vi "mobileyepaser.vi"() -> (2 "headway time":dbl)   [LabVIEW 2015]
uses:
  G_LCM.vi
  G_SEN.vi
panel:
  out "Array":dbl[][](array[numeric])
  out "vel":dbl
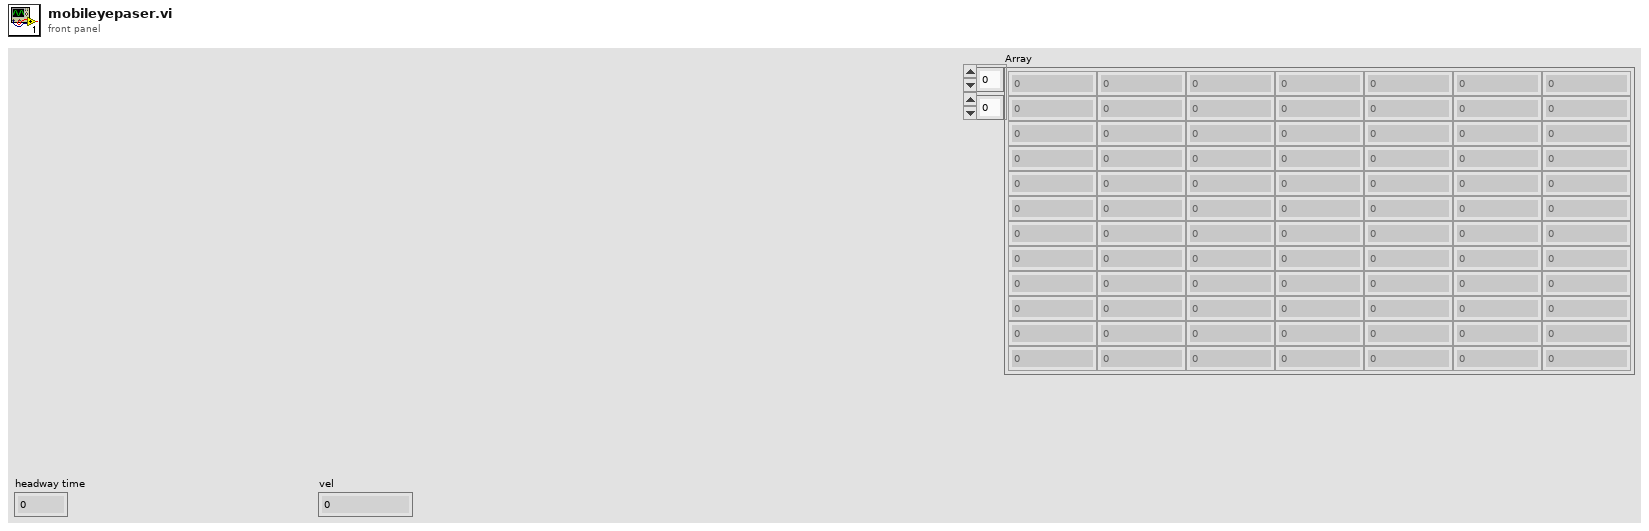
[diagram p1: front panel]
types:
  T1 = cluster{"hash":i64, "sys time":i64, "mobileye":u8[]}
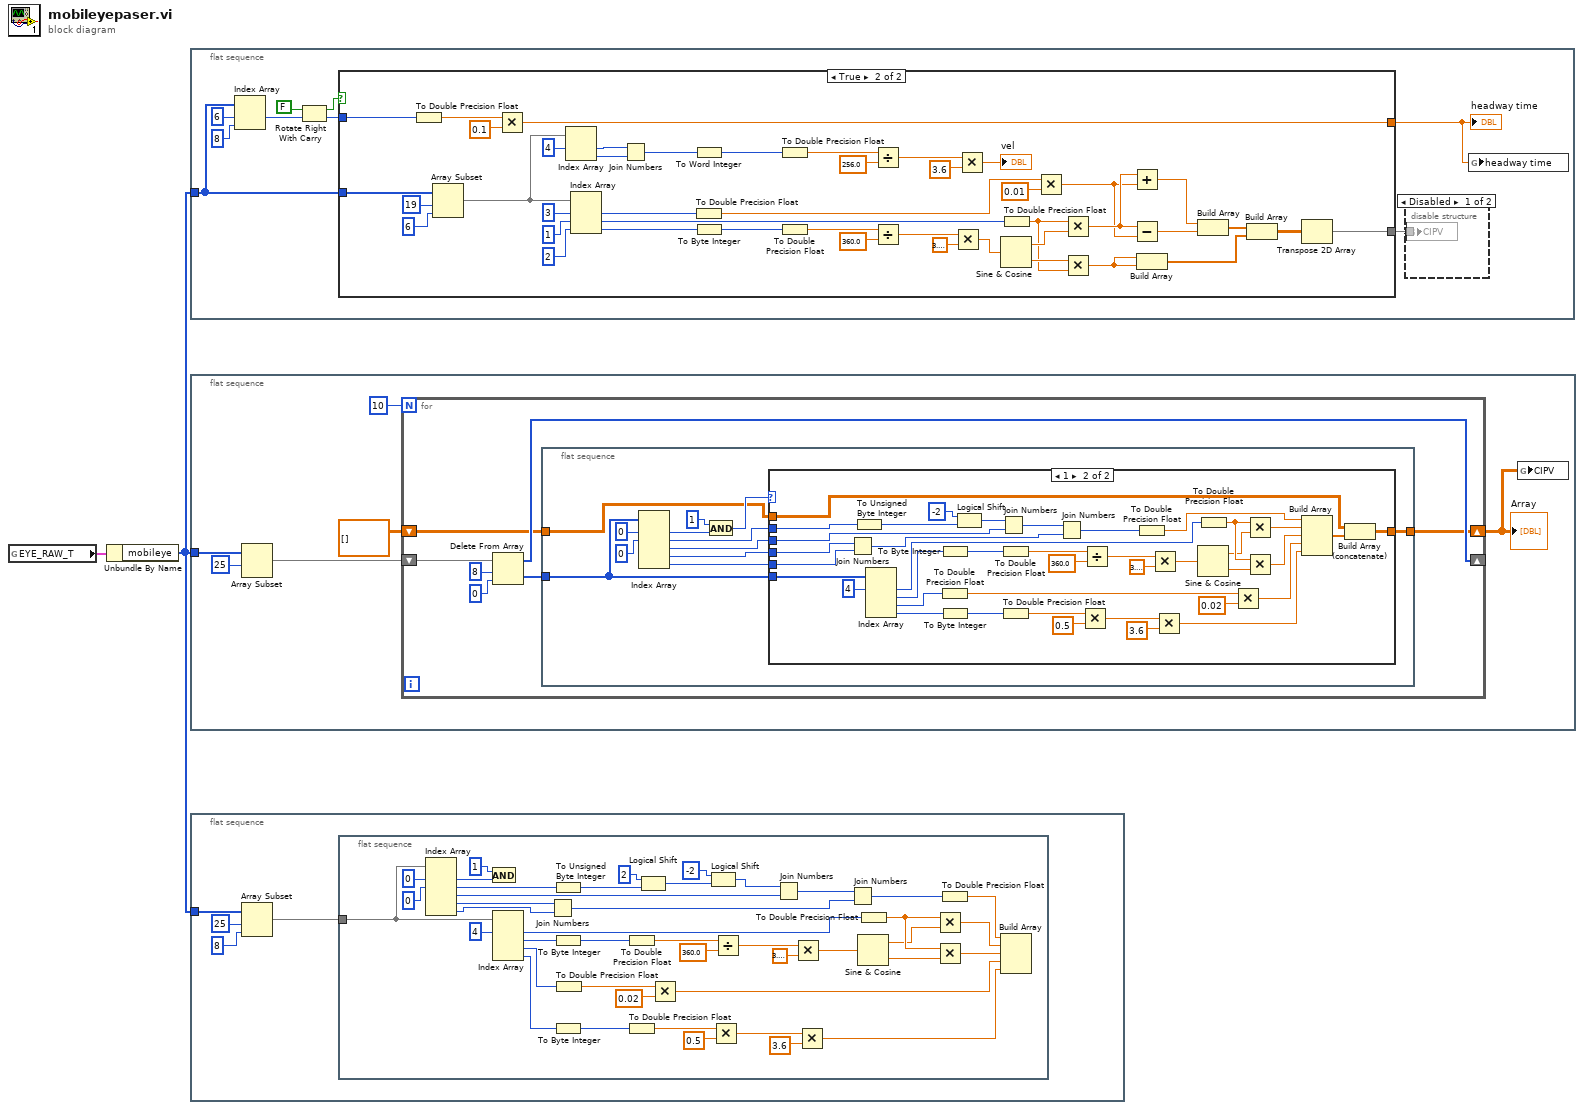
[diagram p0: block diagram]
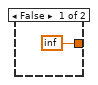
[diagram p4: hidden frame]
diagram:
  n1 = global read "G_LCM.vi" "EYE_RAW_T"() -> (w2:T1)
  n2 = Unbundle By Name(w2) -> ("mobileye"=w1:u8[])
  n3 = flat-sequence {
    tunnel: w1 -> [w5]
    frame #0 {
      n4 = Index Array(array=w5, index #1=6 ("index"), index #2=8 ("index")) -> (element #1=w9:u8)  [unwired: 1 out]
      n5 = Rotate Right With Carry(2:w9, 3:FALSE ("carry")) -> (0:w7:u8, 1:w6:bool)
      n6 = case shown="True" w6 {
        tunnel: w7 -> [_ w28]
        tunnel: [inf w27] -> w3
        tunnel: w5 -> [_ w57]
        tunnel: [_ w31] -> w4
        frame False {
        }
        frame True {
          n7 = To Double Precision Float(number=w28) -> (double precision float=w30:dbl)
          n8 = Array Subset(array=w57, index=19, length=6) -> (w26:u8[])
          n9 = Multiply(x=w30, y=0.1) -> (x*y=w27:dbl)
          n10 = Index Array(array=w26, index #1=4 ("index")) -> (element #1=w48:u8, element #2=w47:u8)  [unwired: 1 in]
          n11 = Index Array(array=w26, index #1=3 ("index"), index #2=1 ("index"), index #3=2 ("index")) -> (element #1=w24:u8, element #2=w18:u8, element #3=w22:u8)
          n12 = Join Numbers(hi=w48, lo=w47) -> ((hi.lo)=w16:u16)
          n13 = To Word Integer(number=w16) -> (16bit integer=w15:i16)
          n14 = To Double Precision Float(number=w24) -> (double precision float=w23:dbl)
          n15 = To Byte Integer(number=w22) -> (8bit integer=w21:i8)
          n16 = To Double Precision Float(number=w15) -> (double precision float=w46:dbl)
          n17 = To Double Precision Float(number=w21) -> (double precision float=w20:dbl)
          n18 = Divide(x=w46, y=256.0) -> (x/y=w44:dbl)
          n19 = Divide(x=w20, y=360.0) -> (x/y=w52:dbl)
          n20 = Multiply(x=w52, y=3.141592653589793) -> (x*y=w42:dbl)
          n21 = Multiply(x=w44, y=3.6) -> (x*y=→"vel":dbl)
          n22 = Sine & Cosine(0:w42) -> (1:w41:dbl, 2:w40:dbl)
          n23 = To Double Precision Float(number=w18) -> (double precision float=w17:dbl)
          n24 = Multiply(x=w23, y=0.01) -> (x*y=w38:dbl)
          n25 = Multiply(x=w17, y=w41) -> (x*y=w39:dbl)
          n26 = Multiply(x=w40, y=w17) -> (x*y=w35:dbl)
          n27 = Add(x=w39, y=w38) -> (x+y=w37:dbl)
          n28 = Subtract(x=w39, y=w38) -> (x-y=w36:dbl)
          n29 = Build Array(w35, w35) -> (w33:dbl[])
          n30 = Build Array(w37, w36) -> (w34:dbl[])
          n31 = Build Array(w34, w33) -> (w32:dbl[][])
          n32 = Transpose 2D Array(2D array=w32) -> (transposed array=w31:dbl[][])
        }
      }
      "headway time" <- w3
      n33 = disable-structure shown="Disabled" {
        disable-tunnel: w4 -> [w12 _]
        frame Disabled {
          n34 = global write "G_SEN.vi" "CIPV"(w12) -> ()
        }
        frame Enabled {
        }
      }
      n35 = global write "G_SEN.vi" "headway time"(w3) -> ()
    }
  }
  n36 = flat-sequence {
    tunnel: w1 -> [w63]
    frame #0 {
      n37 = Array Subset(array=w63, index=25) -> (w61:u8[])  [unwired: 1 in]
      n38 = for {
        N: 10 -> [_]
        shift-right: [w69] -> _
        shift-left: w61 -> [w70]
        shift-right: [w65] -> w58
        shift-left: dbl[][] [] -> [w64]
        n39 = Delete From Array(array=w70, length=8, index=0) -> (deleted portion=w66:u8[], array with subset deleted=w69:u8[])
        n40 = flat-sequence {
          tunnel: w66 -> [w82]
          tunnel: [w72] -> w65
          tunnel: w64 -> [w71]
          frame #0 {
            n41 = Index Array(array=w82, index #1=0 ("index"), index #2=0 ("index")) -> (element #1=w74:u8, element #2=w80:u8, element #3=w79:u8, element #4=w78:u8, element #5=w77:u8)  [unwired: 3 in]
            n42 = And(x=u8 1 ("y"), y=w74) -> (x .and. y?=w73:u8)
            n43 = case shown="1" w73 {
              tunnel: w82 -> [_ w109]
              tunnel: w80 -> [_ w106]
              tunnel: w79 -> [_ w105]
              tunnel: w78 -> [_ w104]
              tunnel: w77 -> [_ w103]
              tunnel: [w83 w86] -> w72
              tunnel: w71 -> [w83 w85]
              frame 0, Default {
              }
              frame 1 {
                n44 = Join Numbers(hi=w104, lo=w103) -> ((hi.lo)=w101:u16)
                n45 = To Unsigned Byte Integer(number=w106) -> (unsigned 8bit integer=w108:u8)
                n46 = Index Array(array=w109, index #1=4 ("index")) -> (element #1=w122:u8, element #2=w113:u8, element #3=w121:u8, element #4=w112:u8)  [unwired: 3 in]
                n47 = To Byte Integer(number=w113) -> (8bit integer=w115:i8)
                n48 = To Double Precision Float(number=w121) -> (double precision float=w120:dbl)
                n49 = To Byte Integer(number=w112) -> (8bit integer=w111:i8)
                n50 = Logical Shift(y=i16 -2, x=w108) -> (x << y=w84:u8)
                n51 = Join Numbers(hi=w84, lo=w105) -> ((hi.lo)=w102:u16)
                n52 = To Double Precision Float(number=w115) -> (double precision float=w114:dbl)
                n53 = To Double Precision Float(number=w111) -> (double precision float=w95:dbl)
                n54 = Join Numbers(hi=w102, lo=w101) -> ((hi.lo)=w100:u32)
                n55 = Multiply(x=w95, y=0.5) -> (x*y=w93:dbl)
                n56 = Divide(x=w114, y=360.0) -> (x/y=w117:dbl)
                n57 = To Double Precision Float(number=w100) -> (double precision float=w92:dbl)
                n58 = Multiply(x=w117, y=3.141592653589793) -> (x*y=w99:dbl)
                n59 = Multiply(x=w93, y=3.6) -> (x*y=w88:dbl)
                n60 = Sine & Cosine(0:w99) -> (1:w97:dbl, 2:w96:dbl)
                n61 = To Double Precision Float(number=w122) -> (double precision float=w98:dbl)
                n62 = Multiply(x=w120, y=0.02) -> (x*y=w89:dbl)
                n63 = Multiply(x=w98, y=w97) -> (x*y=w91:dbl)
                n64 = Multiply(x=w98, y=w96) -> (x*y=w90:dbl)
                n65 = Build Array(w92, w91, w90, w89, w88) -> (w87:dbl[])
                n66 = Build Array (concatenate)(w85, w87) -> (w86:dbl[][])
              }
            }
          }
        }
      }
      "Array" <- w58
      n67 = global write "G_SEN.vi" "CIPV"(w58) -> ()
    }
  }
  n68 = flat-sequence {
    tunnel: w1 -> [w127]
    frame #0 {
      n69 = Array Subset(array=w127, index=25, length=8) -> (w124:u8[])
      n70 = flat-sequence {
        tunnel: w124 -> [w156]
        frame #0 {
          n71 = Index Array(array=w156, index #1=0 ("index"), index #2=0 ("index")) -> (element #1=w134:u8, element #2=w152:u8, element #3=w151:u8, element #4=w150:u8, element #5=w149:u8)  [unwired: 3 in]
          n72 = And(x=u8 1 ("y"), y=w134) -> ()  [unwired: 1 out]
          n73 = Index Array(array=w156, index #1=4 ("index")) -> (element #1=w169:u8, element #2=w160:u8, element #3=w168:u8, element #4=w159:u8)  [unwired: 3 in]
          n74 = Join Numbers(hi=w150, lo=w149) -> ((hi.lo)=w147:u16)
          n75 = To Unsigned Byte Integer(number=w152) -> (unsigned 8bit integer=w154:u8)
          n76 = To Byte Integer(number=w160) -> (8bit integer=w162:i8)
          n77 = To Byte Integer(number=w159) -> (8bit integer=w158:i8)
          n78 = To Double Precision Float(number=w168) -> (double precision float=w167:dbl)
          n79 = To Double Precision Float(number=w162) -> (double precision float=w161:dbl)
          n80 = To Double Precision Float(number=w158) -> (double precision float=w138:dbl)
          n81 = Logical Shift(y=i16 2, x=w154) -> (x << y=w145:u8)
          n82 = Multiply(x=w167, y=0.02) -> (x*y=w129:dbl)
          n83 = Logical Shift(y=i16 -2, x=w145) -> (x << y=w139:u8)
          n84 = Multiply(x=w138, y=0.5) -> (x*y=w136:dbl)
          n85 = Divide(x=w161, y=360.0) -> (x/y=w164:dbl)
          n86 = Join Numbers(hi=w139, lo=w151) -> ((hi.lo)=w148:u16)
          n87 = Multiply(x=w164, y=3.141592653589793) -> (x*y=w143:dbl)
          n88 = Multiply(x=w136, y=3.6) -> (x*y=w128:dbl)
          n89 = Join Numbers(hi=w148, lo=w147) -> ((hi.lo)=w144:u32)
          n90 = Sine & Cosine(0:w143) -> (1:w141:dbl, 2:w140:dbl)
          n91 = To Double Precision Float(number=w169) -> (double precision float=w142:dbl)
          n92 = Multiply(x=w142, y=w141) -> (x*y=w131:dbl)
          n93 = Multiply(x=w142, y=w140) -> (x*y=w130:dbl)
          n94 = To Double Precision Float(number=w144) -> (double precision float=w132:dbl)
          n95 = Build Array(w132, w131, w130, w129, w128) -> ()  [unwired: 1 out]
        }
      }
    }
  }
